vi "Calibrate Buttons Speed 2 Ticks (uSMC).vi"(6 "Backlash Speed (Full Steps/Sec)":u16, 7 "Reset Speed (Full Steps/Sec)":u16, 8 "Buttons Speed 4 (Full Steps/Sec)":u16, 9 "Buttons Speed 3 (Full Steps/Sec)":u16, 10 "Buttons Speed 2 (Full Steps/Sec)":u16, 11 "Buttons Speed 1 (Full Steps/Sec)":u16) -> (0 "Buttons Speed 4 (ticks)":u16=63573, 1 "Buttons Speed 3 (ticks)":u16=61610, 2 "Buttons Speed 2 (ticks)":u16=55720, 3 "Buttons Speed 1 (ticks)":u16=26270, 4 "Backlash Speed (ticks)":u16, 5 "Reset Speed (ticks)":u16=63573)   [LabVIEW 2010, in "SignalWriterMH110203USBStepperMotor.lvclass"]
uses:
  SignalWriterMH110203USBStepperMotor.lvclass
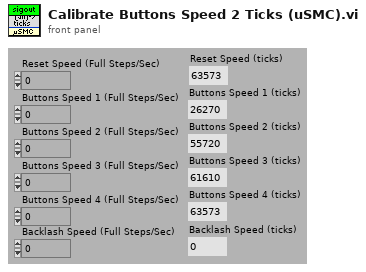
[diagram p1: front panel]
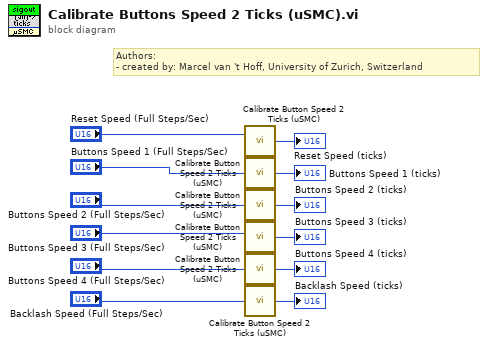
[diagram p0: block diagram]
diagram:
  # "Authors: \n- created by: Marcel van 't Hoff, University of Zurich, Switzerland"
  n1 = call "Calibrate Button Speed 2 Ticks (uSMC).vi"("Speed (Full Step/Sec)"="Reset Speed (Full Steps/Sec)") -> ("Ticks"=→"Reset Speed (ticks)":u16)
  n2 = call "Calibrate Button Speed 2 Ticks (uSMC).vi"("Speed (Full Step/Sec)"="Buttons Speed 1 (Full Steps/Sec)") -> ("Ticks"=→"Buttons Speed 1 (ticks)":u16)
  n3 = call "Calibrate Button Speed 2 Ticks (uSMC).vi"("Speed (Full Step/Sec)"="Buttons Speed 2 (Full Steps/Sec)") -> ("Ticks"=→"Buttons Speed 2 (ticks)":u16)
  n4 = call "Calibrate Button Speed 2 Ticks (uSMC).vi"("Speed (Full Step/Sec)"="Buttons Speed 3 (Full Steps/Sec)") -> ("Ticks"=→"Buttons Speed 3 (ticks)":u16)
  n5 = call "Calibrate Button Speed 2 Ticks (uSMC).vi"("Speed (Full Step/Sec)"="Buttons Speed 4 (Full Steps/Sec)") -> ("Ticks"=→"Buttons Speed 4 (ticks)":u16)
  n6 = call "Calibrate Button Speed 2 Ticks (uSMC).vi"("Speed (Full Step/Sec)"="Backlash Speed (Full Steps/Sec)") -> ("Ticks"=→"Backlash Speed (ticks)":u16)
